vi "New LPS Sensor.vi"(8 "error in (no error)":errorcluster, 10 "I2C Slave Address (0x5D)":u8=93 format="%.0x", 11 "I2C":refnum<class "LINX I2C.lvclass">) -> (0 "error out":errorcluster, 3 "LPS Barometer out":refnum<class "LPS Barometric Pressure Sensor.lvclass">)   [LabVIEW 2020, in "LPS Barometric Pressure Sensor.lvclass"]
doc: "Creates a new LPS25H object from the configured I2C channel."
uses:
  LPS Barometric Pressure Sensor.lvclass
  LINX I2C/LINX I2C.lvclass
panel:
  # "Default = SA0 HIGH \nSA0 LOW = 0b1011100\nSA0 HIGH = 0b1011101"
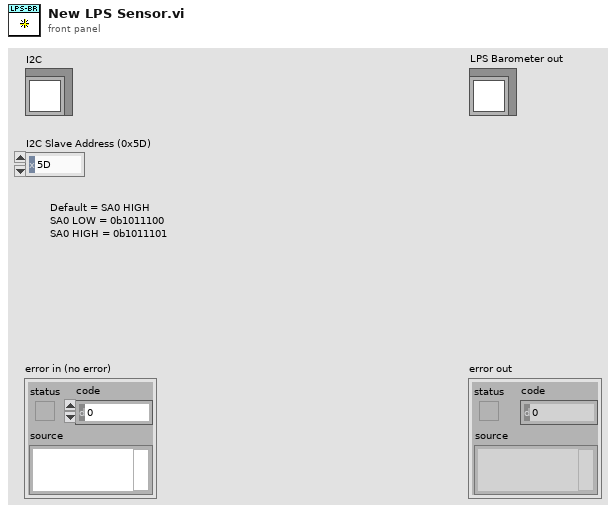
[diagram p1: front panel]
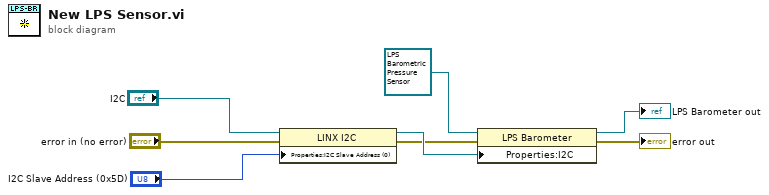
[diagram p0: block diagram]
diagram:
  n1 = property class="LINX I2C"(reference="I2C", error in="error in (no error)", "Properties:I2C Slave Address (0)"="I2C Slave Address (0x5D)") -> (reference out=w5:refnum<class "LINX I2C.lvclass">, error out=w4:errorcluster)
  n2 = property class="LPS Barometer"(reference=refnum<class "LPS Barometric Pressure Sensor.lvclass"> refnum ("LPS Barometer in"), error in=w4, "Properties:I2C"=w5) -> (reference out=→"LPS Barometer out":refnum<class "LPS Barometric Pressure Sensor.lvclass">, error out=→"error out":errorcluster)
